vi "主画面.vi"() -> ()   [LabVIEW 2016]
uses:
  <vilib>/Utility/config.llb/Read Key (String).vi
  <vilib>/Utility/config.llb/NI_LVConfig.lvlib
  data/FreeMem.dll
panel:
  in  "全屏":T1
  out "站点名称":string="站点名称"
  out "时间显示":string="2017-05-09 10:50:42"
  out "Version":string="Version:1.0.0"
  in  "主画面菜单":enum32{"首页", "数据查询", "运维调试", "系统设置"}(xcontrol)
  # "ESTD-XP 一体化水质自动监测系统"
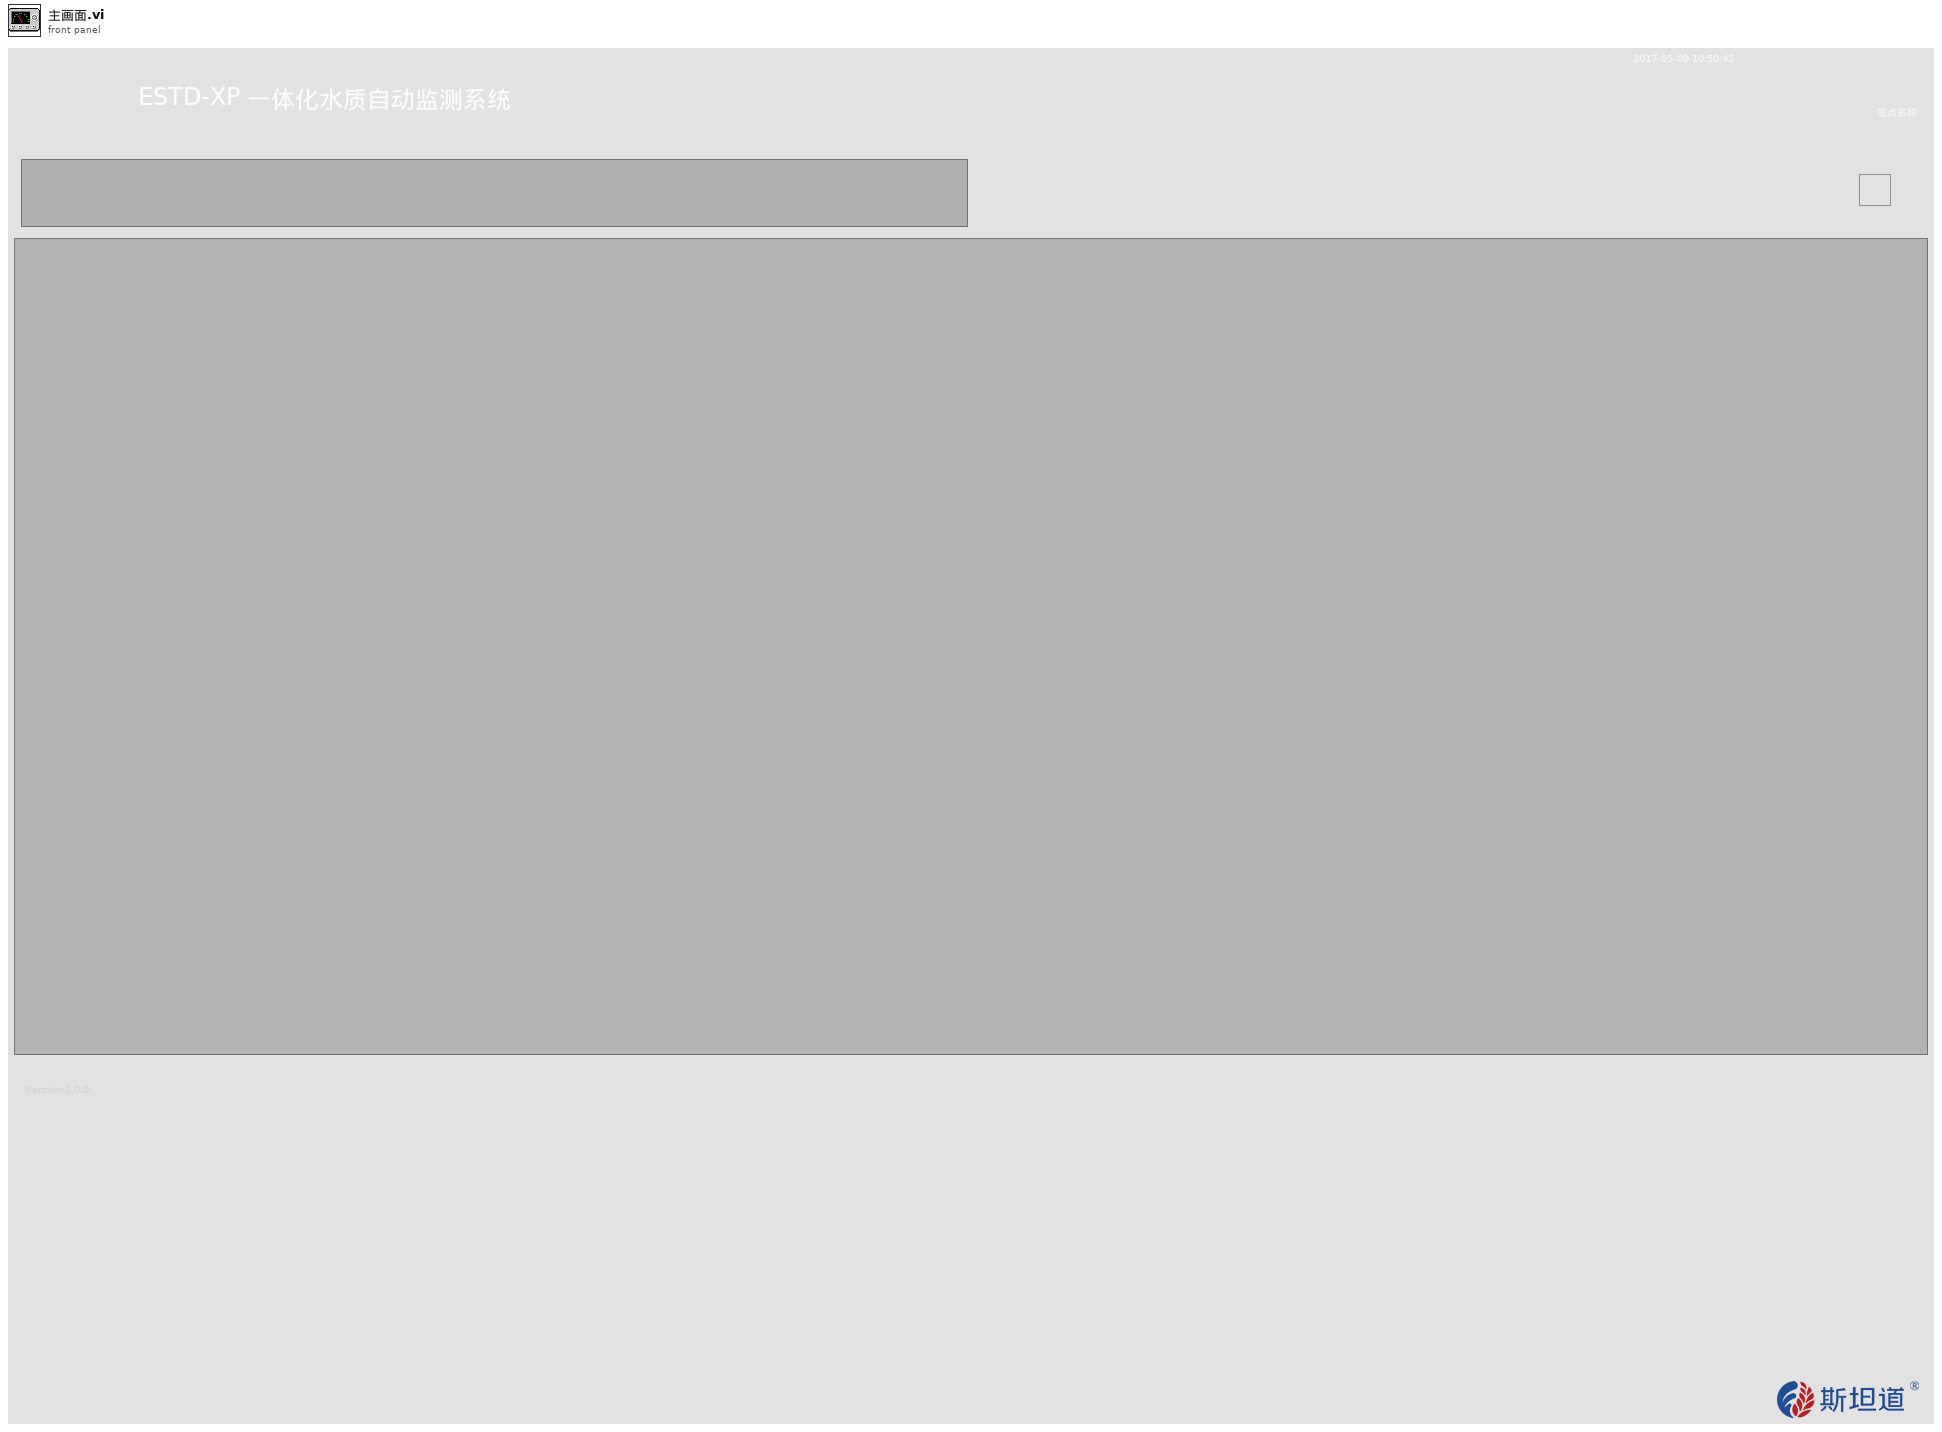
[diagram p1: front panel]
types:
  T1 = typedef "全屏按钮.ctl" = bool
  T2 = cluster{"时间标识":timestamp, "设备":string, "日志信息":string, "流程参数":string}
  T3 = enum32{"invalid app kind", "Development System", "Run Time System", "Student Edition", "Embedded LabVIEW", "Evaluation", "Custom"}
  T4 = typedef "NI_LVConfig.lvlib/Config Data RefNum.ctl" = refnum<k1>
  T5 = enum32{"Bad", "Idle", "Run top level", "Running"}
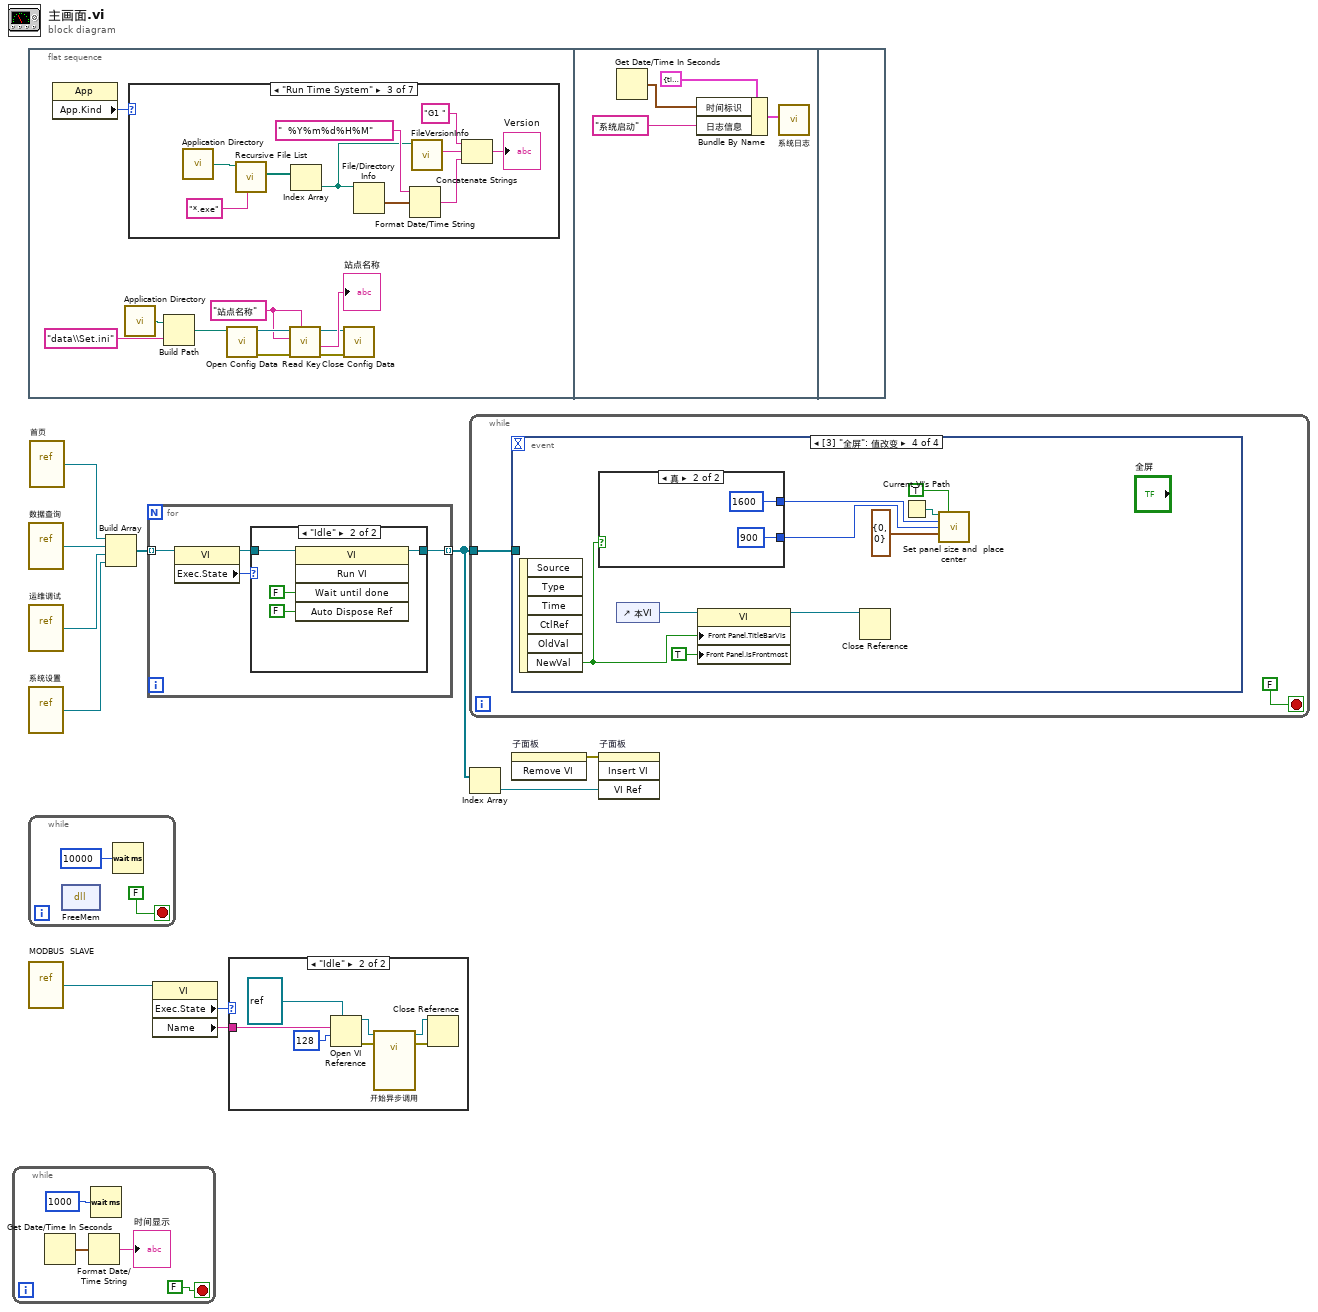
[diagram p0: block diagram]
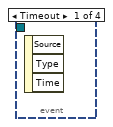
[diagram p10: hidden frame]
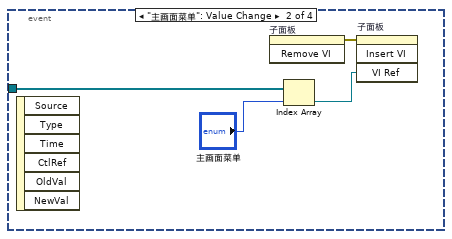
[diagram p11: hidden frame]
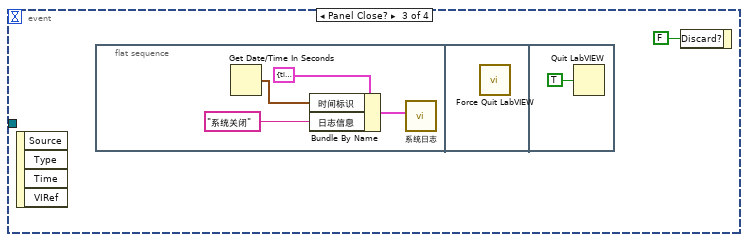
[diagram p12: hidden frame]
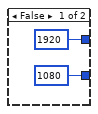
[diagram p13: hidden frame]
diagram:
  n1 = while {
    stop <- FALSE stop-if-true
    n2 = Get Date/Time In Seconds() -> (seconds since 1Jan1904=w12:timestamp)
    n3 = Format Date/Time String(seconds (now)=w12) -> (date/time string=→"时间显示":string)  [unwired: 2 in]
    n4 = Wait (ms)(milliseconds to wait=u32 1000 ("等待时间（毫秒）")) -> ()  [unwired: 1 out]
  }
  n5 = flat-sequence {
    frame #0 {
      w16 = "站点名称" ("section")
      n6 = property class="App"() -> ("App.Kind"=w25:T3)  [unwired: 2 in, 2 out]
      n7 = call <vilib>:"Application Directory.vi"() -> ("Application Directory"=w19:path)
      n8 = case shown="\"Run Time System\"" w25 {
        frame "invalid app kind" {
        }
        frame "Development System", Default {
        }
        frame "Run Time System" {
          n9 = call <vilib>:"Application Directory.vi"() -> ("Application Directory"=w27:path)
          n10 = call <vilib>:"Recursive File List.vi"("pattern"="*.exe", "Folder Path"=w27) -> ("All Files in Dir"=w28:path[])  [unwired: 5 in, 4 out]
          n11 = Index Array(array=w28) -> (element=w26:path)  [unwired: 1 in]
          n12 = File/Directory Info(path=w26) -> (last mod=w32:timestamp)  [unwired: 1 in, 6 out]
          n13 = Format Date/Time String(time format string (%c)="  %Y%m%d%H%M" ("时间格式字符串(%c)"), seconds (now)=w32) -> (date/time string=w30:string)  [unwired: 1 in]
          n14 = call <vilib>:"FileVersionInfo.vi"("Application Path in"=w26) -> ("File Version Info"=w34:string)  [unwired: 7 in, 3 out]
          n15 = Concatenate Strings("G1 " ("字符串"), w34, w30) -> (→"Version":string)
        }
        frame "Student Edition" {
        }
        frame "Embedded LabVIEW" {
        }
        frame "Evaluation" {
        }
        frame "Custom" {
        }
      }
      n16 = Build Path(base path=w19, name or relative path="data\\Set.ini" ("名称或相对路径")) -> (appended path=w17:path)
      n17 = call <vilib>:"Open Config Data.vi"("configuration file path"=w17) -> ("error out"=w21:errorcluster, "refnum"=w24:T4)  [unwired: 8 in, 1 out]
      n18 = call-poly <vilib>:"Read Key.vi"("section"=w16, "error in (no error)"=w21, "key"=w16, "refnum"=w24) -> ("error out"=w20:errorcluster, "value"=→"站点名称":string, "refnum out"=w22:T4)  [unwired: 4 in, 1 out]
      n19 = call <vilib>:"Close Config Data.vi"("error in (no error)"=w20, "refnum"=w22) -> ()  [unwired: 8 in, 2 out]
    }
    frame #1 {
      n20 = Get Date/Time In Seconds() -> (seconds since 1Jan1904=w37:timestamp)
      n21 = Bundle By Name(cluster=T2 {"时间标识"=timestamp(0 s since 1904-01-01), "设备"="系统", "日志信息"="", "流程参数"=""} ("data in"), "时间标识"=w37, "日志信息"="系统启动") -> (w38:T2)
      n22 = call "系统日志.vi"("data in"=w38) -> ()  [unwired: 11 in]
    }
    frame #2 {
    }
  }
  n23 = vi-ref "数据查询.vi"() -> (w7:refnum<vi>)
  n24 = vi-ref "运维调试.vi"() -> (w6:refnum<vi>)
  n25 = vi-ref "系统设置.vi"() -> (w5:refnum<vi>)
  n26 = while {
    stop <- FALSE stop-if-true
    n27 = dll-call lib="PTH2mabs F\tgitkraken集成模板固定站（模板）!一体站项目 - 固定站模板dataFreeMem.dll" fn="FreeMem"() -> ()  [unwired: 4 in, 2 out]
    n28 = Wait (ms)(milliseconds to wait=u32 10000 ("等待时间（毫秒）")) -> ()  [unwired: 1 out]
  }
  n29 = vi-ref "MODBUS  SLAVE.vi"() -> (w3:refnum<vi>)
  n30 = vi-ref "首页.vi"() -> (w8:refnum<vi>)
  n31 = Build Array(w8, w7, w6, w5) -> (w4:refnum<vi>[])
  n32 = for {
    tunnel: w4 -> [w45] mode=indexing
    tunnel: [w42] -> w10 mode=indexing
    n33 = property class="VI"(reference=w45) -> (reference out=w43:refnum<vi>, "Exec.State"=w44:T5)  [unwired: 1 in, 1 out]
    n34 = case shown="\"Idle\"" w44 {
      tunnel: w43 -> [w46 w48]
      tunnel: [w46 w47] -> w42
      frame "Bad", Default {
      }
      frame "Idle" {
        n35 = invoke class="VI" method="Run VI"(reference=w48, "Wait until done"=FALSE ("结束前等待"), "Auto Dispose Ref"=FALSE ("自动销毁引用")) -> (reference out=w47:refnum<vi>)  [unwired: 2 in, 4 out]
      }
    }
  }
  n36 = property class="VI"(reference=w3) -> ("Exec.State"=w2:T5, "Name"=w1:string)  [unwired: 1 in, 2 out]
  n37 = case shown="\"Idle\"" w2 {
    tunnel: w1 -> [_ w51]
    frame "Bad", Default {
    }
    frame "Idle" {
      n38 = Open VI Reference(type specifier VI Refnum (for type only)=refnum<vi> refnum, vi path=w51, options=128 ("选项")) -> (vi reference=w53:refnum<vi>, error out=w56:errorcluster)  [unwired: 3 in]
      n39 = call-by-ref "开始异步调用"(reference=w53, error in=w56) -> (reference out=w55:refnum<vi>, error out=w57:errorcluster)  [unwired: 11 in, 1 out]
      n40 = Close Reference(reference=w55, error in (no error)=w57) -> ()  [unwired: 1 out]
    }
  }
  n41 = while {
    tunnel: w10 -> [w58]
    stop <- FALSE stop-if-true
    n42 = event shown="[3] \"全屏\": 值改变" {
      selector: _ -> [_ _ _ _]
      dyn-events: _ -> [_ _ _ _]
      timeout: _ -> [_ _ _ _]
      tunnel: w58 -> [_ w62 _ _]
      event Timeout {
        n43 = event-data() -> ()  [unwired: 1 in, 3 out]
      }
      event "主画面菜单": Value Change {
        n44 = event-data() -> ()  [unwired: 1 in, 6 out]
        n45 = invoke on="子面板" class="SubPnl" method="Remove VI"() -> (error out=w60:errorcluster)  [unwired: 3 in, 2 out]
        n46 = Index Array(array=w62, index="主画面菜单") -> (element=w61:refnum<vi>)
        n47 = invoke on="子面板" class="SubPnl" method="Insert VI"(error in=w60, "VI Ref"=w61) -> ()  [unwired: 2 in, 4 out]
      }
      event Panel Close? {
        n48 = event-data() -> ()  [unwired: 1 in, 4 out]
        n49 = flat-sequence {
          frame #0 {
            n50 = Get Date/Time In Seconds() -> (seconds since 1Jan1904=w67:timestamp)
            n51 = Bundle By Name(cluster=T2 {"时间标识"=timestamp(0 s since 1904-01-01), "设备"="系统", "日志信息"="", "流程参数"=""} ("data in"), "时间标识"=w67, "日志信息"="系统关闭") -> (w66:T2)
            n52 = call "系统日志.vi"("data in"=w66) -> ()  [unwired: 11 in]
          }
          frame #1 {
            n53 = call "Force Quit LabVIEW.vi"() -> ()  [unwired: 10 in, 2 out]
          }
          frame #2 {
            n54 = Quit LabVIEW(quit? (T)=TRUE ("退出？(T)")) -> ()
          }
        }
        n55 = event-data("Discard?"=FALSE ("放弃？")) -> ()  [unwired: 1 in, 1 out]
      }
      event Value Change {
        n56 = event-data() -> ("NewVal"=w73:T1)  [unwired: 1 in, 5 out]
        n57 = case shown="真" w73 {
          tunnel: [1920 ("Panel Width") 1600 ("Panel Width")] -> w72
          tunnel: [1080 ("Panel Height") 900 ("Panel Height")] -> w71
          frame False {
          }
          frame True {
          }
        }
        n58 = control-ref of="本VI"() -> (w78:refnum<vi>)
        n59 = property class="VI"(reference=w78, "Front Panel.TitleBarVis"=w73, "Front Panel.IsFrontmost"=TRUE ("前面板窗口:在最前")) -> (reference out=w74:refnum<vi>)  [unwired: 1 in, 1 out]
        n60 = Close Reference(reference=w74) -> ()  [unwired: 1 in, 1 out]
        n61 = Current VI's Path() -> (path=w77:path)
        n62 = call "Set panel size and  place center.vi"("Path"=w77, "Close Reference (false)"=TRUE, "Panel Width"=w72, "Panel Height"=w71, "FP.Origin in(H & V)"=cluster{"Horizontal":i16, "Vertical":i16} {"Horizontal"=0, "Vertical"=0}) -> ()  [unwired: 6 in, 5 out]
      }
    }
  }
  n63 = Index Array(array=w10) -> (element=w9:refnum<vi>)  [unwired: 1 in]
  n64 = invoke on="子面板" class="SubPnl" method="Remove VI"() -> (error out=w11:errorcluster)  [unwired: 3 in, 2 out]
  n65 = invoke on="子面板" class="SubPnl" method="Insert VI"(error in=w11, "VI Ref"=w9) -> ()  [unwired: 2 in, 4 out]
